vi "Module Name--constant.vi"() -> (3 "Module Name":string)   [LabVIEW 2025, in "Central Monitor.lvlib"]
doc: "Return the name of the module that owns this VI. \n_____\nBased on DQMH Dev Tools: Project Template 7.1.2.1547."
uses:
  Central Monitor.lvlib
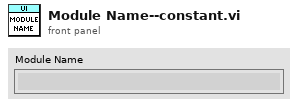
[diagram p1: front panel]
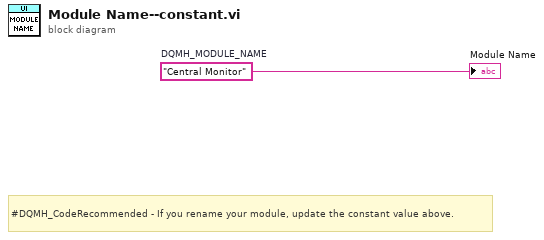
[diagram p0: block diagram]
diagram:
  w1 = "Central Monitor"  # DQMH_MODULE_NAME
  # "#DQMH_CodeRecommended - If you rename your module, update the constant value above."
  "Module Name" <- w1
